vi "CM-BOOL Obstacle.vi"(1 "Threshold":dbl, 2 "Value":sgl) -> (0 "Obstacle??":bool)   [LabVIEW 2015]
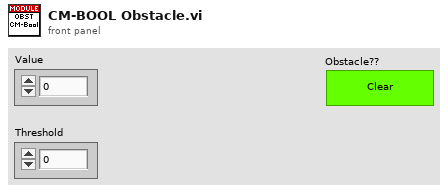
[diagram p1: front panel]
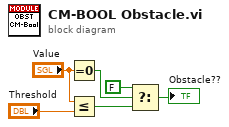
[diagram p0: block diagram]
diagram:
  n1 = Equal To 0?(x="Value") -> (x = 0?=w5:bool)
  n2 = Less Or Equal?(x="Value", y="Threshold") -> (x <= y?=w4:bool)
  n3 = Select(t=FALSE, s=w5, f=w4) -> (s? t:f=→"Obstacle??":bool)
